vi "lab_3_14.vi"() -> ()   [LabVIEW 2014]
uses:
  <vilib>/measure/NI_MABase.lvlib
  <vilib>/addons/Multicore Analysis and Sparse Matrix/Statistics/NI_MASM_Statistics.lvlib
  <vilib>/addons/Multicore Analysis and Sparse Matrix/Statistics/_statistics/Mean (DBL).vi
panel:
  in  "frequency quadra":dbl=10.0 format="%0.2p"
  in  "tempo tot acquisiz":dbl=10.0
  in  "durata ciclo\n acquisizione dt":dbl=0.1
  in  "freq acquiisizione":dbl=100.0
  out "XY Graph":cluster{dbl[], dbl[]}(graph)={[0.0, 0.1, 0.2, 0.30000000000000004, 0.4, 0.5, 0.6000000000000001, 0.7000000000000001, 0.8, 0.9, 1.0, 1.1, 1.2000000000000002, 1.3, 1.4000000000000001, 1.5, 1.6, 1.7000000000000002, 1.8, 1.9000000000000001, 2.0, 2.1, 2.2], [-0.6283331725440203, -0.6232331428373039, -0.6252402512745634, -0.6234305633482926, -0.6236608872729936, -0.6242860521993236, -0.6224763642290302, -0.6245163760942043, -0.625503478609293, -0.6266880016278467, -0.6394545275464434, -0.6367235438716996, -0.6305706048010584, -0.6251086375340427, -0.6216537787404632, -0.6258325127301287, -0.6230357222540388, -0.618824084876408, -0.617080203781738, -0.6219170060895249, -0.6277738143470255, -0.6266221947287355, -0.6307680253237332]}
  in  "amp quadra":dbl=1.0 format="%0.2p"
  out "Waveform Graph 2":waveform(dbl)(graph)={"t0"=timestamp(0 s since 1904-01-01), "dt"=0.001, "Y"=array[1000 elements]}
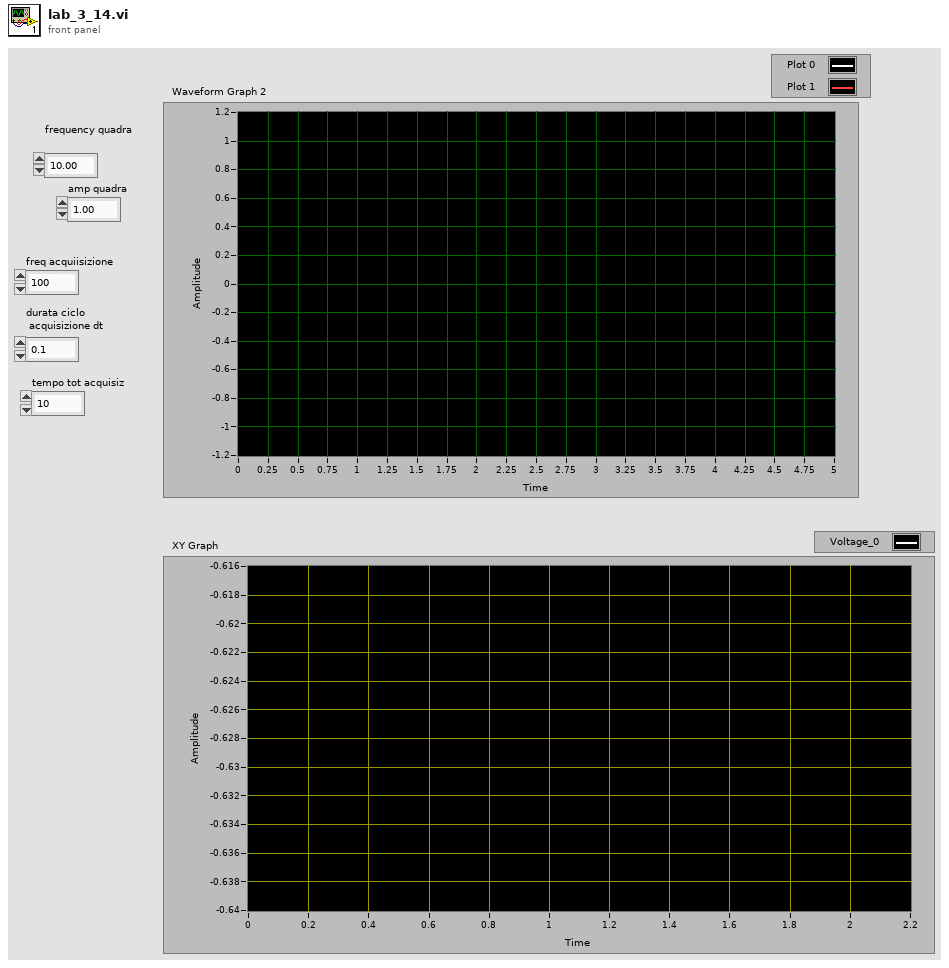
[diagram p1: front panel]
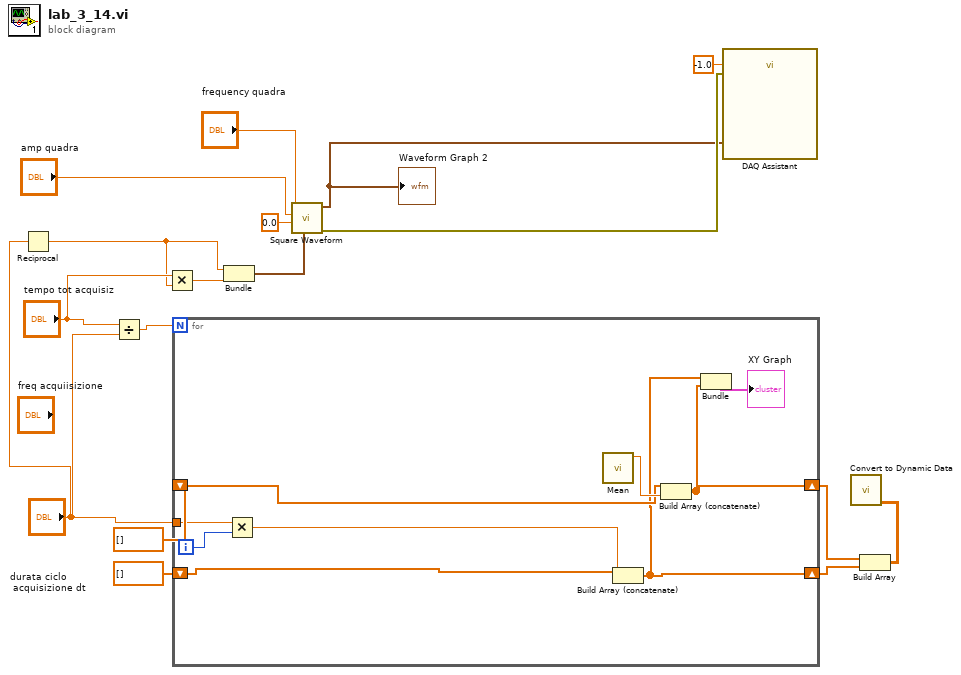
[diagram p0: block diagram]
diagram:
  n1 = Reciprocal(x="durata ciclo\n acquisizione dt") -> (1/x=w3:dbl)
  n2 = Divide(x="tempo tot acquisiz", y="durata ciclo\n acquisizione dt") -> (x/y=w15:dbl)
  n3 = Multiply(x="tempo tot acquisiz", y=w3) -> (x*y=w2:dbl)
  n4 = for {
    N: w15 -> [_]
    shift-right: [w19] -> w12
    shift-left: dbl[] [] -> [w25]
    tunnel: "durata ciclo\n acquisizione dt" -> [w20]
    shift-right: [w18] -> w11
    shift-left: dbl[] [] -> [w22]
    i -> [w24]
    n5 = Multiply(x=w20, y=w24) -> (x*y=w23:dbl)
    n6 = call-poly <vilib>:"Mean.vi"() -> ("mean"=w26:dbl)  [unwired: 10 in, 1 out]
    n7 = Build Array (concatenate)(w22, w23) -> (w18:dbl[])
    n8 = Build Array (concatenate)(w25, w26) -> (w19:dbl[])
    n9 = Bundle(w18, w19) -> (→"XY Graph":cluster{dbl[], dbl[]})  [unwired: 1 in]
  }
  n10 = Bundle(w3, w2) -> (w5:cluster{dbl, dbl})  [unwired: 1 in]
  n11 = call <vilib>:"Square Waveform.vi"("sampling info"=w5, "phase"=0.0, "amplitude"="amp quadra", "frequency"="frequency quadra") -> ("error out"=w9:errorcluster, "signal out"=w6:waveform(dbl))  [unwired: 6 in]
  "Waveform Graph 2" <- w6
  n12 = call "DAQ Assistant"("data"=w6, "timeout (s)"=-1.0, "error in"=w9) -> ()  [unwired: 15 in, 2 out]
  n13 = Build Array(w12, w11) -> (w10:dbl[][])
  n14 = call "Convert to Dynamic Data"("2D Array"=w10) -> ()  [unwired: 3 in, 1 out]
